vi "Open Bitfile.vi"(8 "error in (no error)":errorcluster, 9 "Bitfile path":path) -> (0 "error out":errorcluster, 1 "Interface Out":T1)   [LabVIEW 2015]
uses:
  TypeDefs Host/FPGA Dynamic Interface.ctl
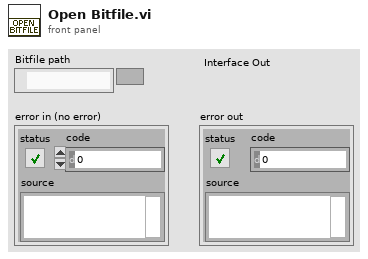
[diagram p1: front panel]
types:
  T1 = typedef "FPGA Dynamic Interface.ctl" = refnum<k20>
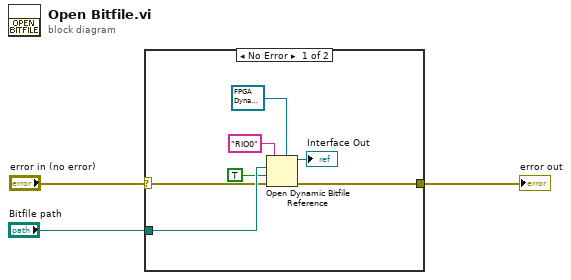
[diagram p0: block diagram]
diagram:
  n1 = case shown="No Error" "error in (no error)" {
    selector: "error in (no error)" -> [w6 w11]
    tunnel: "Bitfile path" -> [w10 _]
    tunnel: [w7 w11] -> w2
    frame No Error {
      n2 = Open Dynamic Bitfile Reference(0:"RIO0" ("Device address"), 1:w10, 2:TRUE, 3:w6, 4:T1 refnum ("Dynamic Ref In")) -> (5:→"Interface Out":T1, 8:w7:errorcluster)
    }
    frame Error {
    }
  }
  "error out" <- w2
